vi "FTW-Endpoint-Multipart-Tell.vi"(0 "FTW Endpoint":refnum<class "FTW-Endpoint-TCP.lvclass">, 5 "Message":T1, 7 "Timeout":i32 format="%dmsec", 11 "error in":errorcluster) -> (4 "FTW Endpoint out":refnum<class "FTW-Endpoint-TCP.lvclass">, 6 "Timed out?":bool, 15 "error out":errorcluster)   [LabVIEW 2013, in "FTW-Endpoint-TCP.lvclass"]
uses:
  FTW-Endpoint-TCP.lvclass
  Payload/FTW-MessagePayload.ctl
panel:
  # "Inputs"
  # "Outputs"
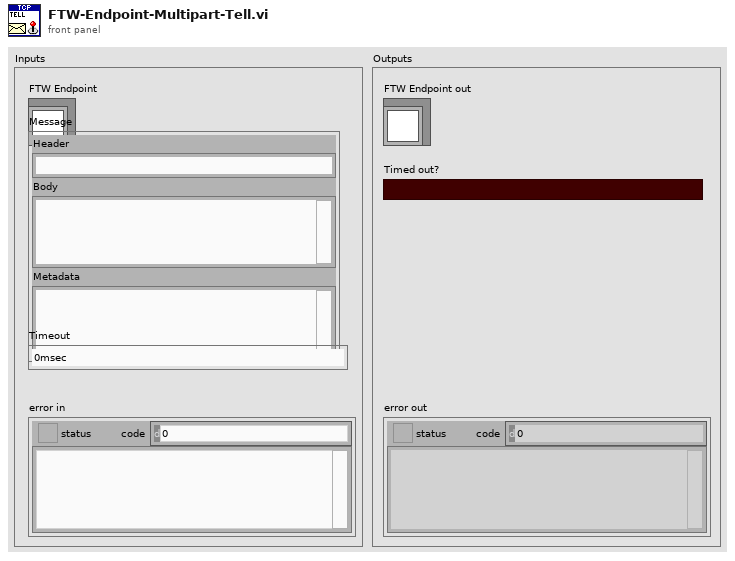
[diagram p1: front panel]
types:
  T1 = typedef "FTW-MessagePayload.ctl" = cluster{"Header":string, "Body":string, "Metadata":string}
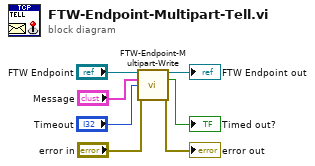
[diagram p0: block diagram]
diagram:
  n1 = call-dynamic "FTW-Endpoint-Multipart-Write.vi"("FTW Endpoint"="FTW Endpoint", "Message"="Message", "Timeout"="Timeout", "error in"="error in") -> ("FTW Endpoint out"=→"FTW Endpoint out":refnum<class "FTW-Endpoint-TCP.lvclass">, "Timed out?"=→"Timed out?":bool, "error out"=→"error out":errorcluster)  [unwired: 9 in]
